vi "Sort Histogram Data.vi"(11 "Data":variant) -> (1 "Array 2":bool[](array[boolean]), 2 "Array 3":bool[](array[boolean]), 3 "XY Graph":cluster{i32, "Histogram Data":i16}[](graph), 4 "Array":bool[](array[boolean]), 5 "File Path":path)   [LabVIEW 2017]
panel:
  out "Sensor Data":i32[](array[numeric])
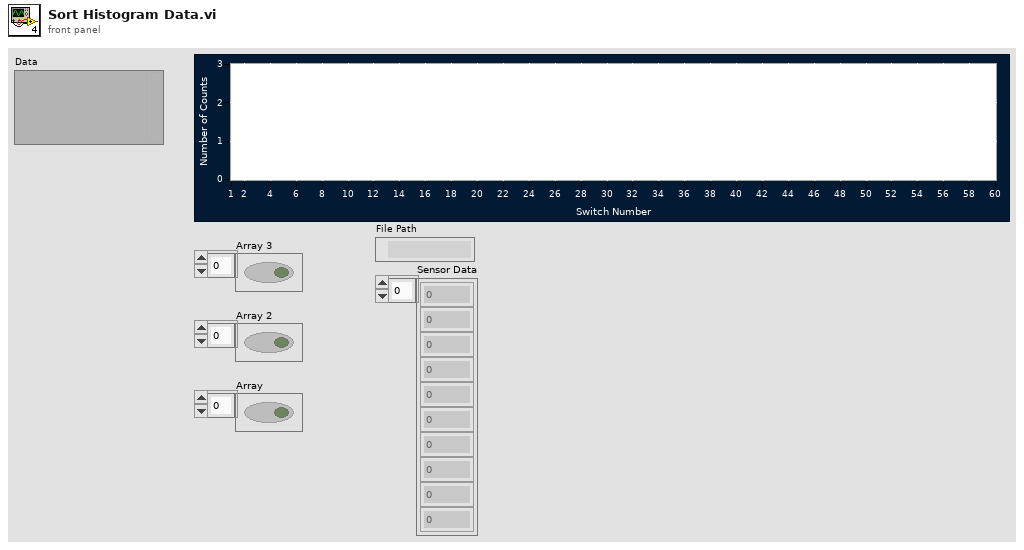
[diagram p1: front panel]
types:
  T1 = cluster{"Histogram Data":i16[], "Sensor Data":i16[], "File Path":path}
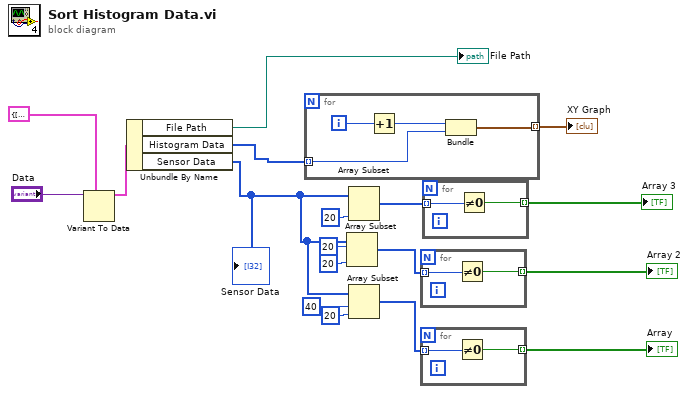
[diagram p0: block diagram]
diagram:
  n1 = Variant To Data(type=T1 {"Histogram Data"=[], "Sensor Data"=[], "File Path"=path ""}, Variant="Data") -> (data=w5:T1)  [unwired: 1 in, 1 out]
  n2 = Unbundle By Name(w5) -> ("File Path"=→"File Path":path, "Histogram Data"=w4:i16[], "Sensor Data"=w3:i16[])
  "Sensor Data" <- w3
  n3 = for {
    tunnel: [w22] -> w7 mode=indexing
    tunnel: w4 -> [w19] mode=indexing
    i -> [w21]
    n4 = Increment(x=w21) -> (x+1=w20:i32)
    n5 = Bundle(w20, "Histogram Data"=w19) -> (w22:cluster{i32, "Histogram Data":i16})  [unwired: 1 in]
  }
  "XY Graph" <- w7
  n6 = Array Subset(array=w3, index=20, length=20) -> (w14:i16[])
  n7 = Array Subset(array=w3, length=20) -> (w13:i16[])  [unwired: 1 in]
  n8 = Array Subset(array=w3, index=40, length=20) -> (w17:i16[])
  n9 = for {
    tunnel: w14 -> [w24] mode=indexing
    tunnel: [w23] -> w16 mode=indexing
    n10 = Not Equal To 0?(x=w24) -> (x != 0?=w23:bool)
  }
  "Array 2" <- w16
  n11 = for {
    tunnel: w17 -> [w26] mode=indexing
    tunnel: [w25] -> w18 mode=indexing
    n12 = Not Equal To 0?(x=w26) -> (x != 0?=w25:bool)
  }
  "Array" <- w18
  n13 = for {
    tunnel: w13 -> [w28] mode=indexing
    tunnel: [w27] -> w15 mode=indexing
    n14 = Not Equal To 0?(x=w28) -> (x != 0?=w27:bool)
  }
  "Array 3" <- w15
